vi "SP Get CH Controls.vi"(5 "S Parameter Test Parameters":T8={"Stimulus"={"Use Instrument Settings"=FALSE, "Blank Frequencies"=FALSE, "Sweep Type"=enum."Linear", "Sweep"={"Fstart"=500.0, "Fstop"=1500.0, "Units"=enum."MHz", "Points"=2}, "Power (dBm)"=999.0, "IFBW (Hz)"=-1.0, "Sweep Time (s)"=-1.0, "Calibration"={"State"=FALSE, "String"=""}}, "Measurement"={"Auto Select"=TRUE, "Data Source"=enum."VNA", "Ports"=2, "Parameters"=[]}, "De-Embed"={"De-Embed"=FALSE, "Adapters"=[]}, "Display"={"Lock Control"=FALSE, "Retain Settings"=TRUE, "Formatted Data"=FALSE, "Plot Orientation"=enum."Single", "Plot Controls"=[{"Trace Orientation"=enum."Overlay", "Frequency"={"Change Frequency"=FALSE, "Start"=500.0, "Stop"=1500.0, "Units"=enum."MHz"}, "Markers"=[], "Traces"=[]}, {"Trace Orientation"=enum."Overlay", "Frequency"={"Change Frequency"=FALSE, "Start"=500.0, "Stop"=1500.0, "Units"=enum."MHz"}, "Markers"=[], "Traces"=[]}, {"Trace Orientation"=enum."Overlay", "Frequency"={"Change Frequency"=FALSE, "Start"=500.0, "Stop"=1500.0, "Units"=enum."MHz"}, "Markers"=[], "Traces"=[]}, {"Trace Orientation"=enum."Overlay", "Frequency"={"Change Frequency"=FALSE, "Start"=500.0, "Stop"=1500.0, "Units"=enum."MHz"}, "Markers"=[], "Traces"=[]}]}, "Limits"=[], "Filter Limits"=[]} {"Filter Limits"."Parameter"."Stimulus Port" min=1 step=1; "Filter Limits"."Parameter"."Response Port" min=1 step=1; "Filter Limits"."Passband"."Bandwidth Attn" format="%.3g"; "Filter Limits"."Passband"."Stop/Span" format="%.3g"; "Filter Limits"."Passband"."Start/Center" format="%.3g"; "Measurement"."Parameters"."Channel" min=0 max=32 step=1; "Measurement"."Parameters"."Parameter"."Stimulus Port" min=1 step=1; "Measurement"."Parameters"."Parameter"."Response Port" min=1 step=1; "Limits"."Parameter"."Stimulus Port" min=1 step=1; "Limits"."Parameter"."Response Port" min=1 step=1; "Stimulus"."Sweep Time (s)" format="%.3g"; "Display"."Plot Controls"."Traces"."Reference" format="%#.2g"; "Display"."Plot Controls"."Traces"."Display Data" items=["Data", "Memory", "Data/Memory"]; "Display"."Plot Controls"."Traces"."Format" items=["Log Mag", "Phase", "Expanded Phase", "Delay", "Smith", "Polar", "Lin Mag", "SWR", "Loss", "Real", "Imaginary"]; "Display"."Plot Controls"."Traces"."Scale" min=0.001 step=1.0 format="%#.2g"; "Display"."Plot Controls"."Traces"."Position" min=0.0 max=10.0; "Display"."Plot Controls"."Frequency"."Stop" format="%.3g"; "Display"."Plot Controls"."Frequency"."Start" format="%.3g"}, 6 "Channel":i8=1, 7 "Plot Reference":refnum<vi>) -> (0 "Channel Control":T5={"Trace On"=TRUE, "Measure"=0, "Format"=0, "Autoscale"=TRUE, "Reference"=0.0, "\nRefUnit"="dB/Div", "Position"=5.0, "Scale"=10.0, "ScaleUnit"="dB/Div", "LimitOn"=TRUE, "LimitFill"=FALSE, "Display Data"=0, "Show Markers"=TRUE, "SXX"=""} {"Reference" format="%#.2g"; "Display Data" items=["Data", "Memory", "Data/Memory"]; "Format" items=["Log Mag", "Phase", "Expanded Phase", "Delay", "Smith", "Polar", "Lin Mag", "SWR", "Loss", "Real", "Imaginary"]; "Scale" min=0.001 step=1.0 format="%#.2g"; "Position" min=0.0 max=10.0}, 1 "CH Controls":T1={"Trace Orientation"=enum."Overlay", "Frequency"={"Change Frequency"=FALSE, "Start"=500.0, "Stop"=1500.0, "Units"=enum."MHz"}, "Markers"=[], "Traces"=[]} {"Traces"."Reference" format="%#.2g"; "Traces"."Display Data" items=["Data", "Memory", "Data/Memory"]; "Traces"."Format" items=["Log Mag", "Phase", "Expanded Phase", "Delay", "Smith", "Polar", "Lin Mag", "SWR", "Loss", "Real", "Imaginary"]; "Traces"."Scale" min=0.001 step=1.0 format="%#.2g"; "Traces"."Position" min=0.0 max=10.0; "Frequency"."Stop" format="%.3g"; "Frequency"."Start" format="%.3g"}, 4 "CH Controls Index":i8)   [LabVIEW 2011]
uses:
  TypeDefs/SP Display Trace Controls.ctl
  TypeDefs/SP Display Format.ctl
  TypeDefs/SP Display Data.ctl
  TypeDefs/SP Test Parameters.ctl
  TypeDefs/SP Stimulus Parameters.ctl
  TypeDefs/SP Frequency Units.ctl
  TypeDefs/SP Calibration State.ctl
  TypeDefs/SP Measurement.ctl
  TypeDefs/SP Parameters.ctl
  TypeDefs/SP Parameter.ctl
  TypeDefs/SP De-Embed.ctl
  TypeDefs/SP Adapter.ctl
  TypeDefs/SP Data.ctl
  TypeDefs/SP Display Parameters.ctl
  TypeDefs/SP Display Plot Controls Cluster.ctl
  TypeDefs/SP Marker Cluster.ctl
  TypeDefs/SP Marker Type.ctl
  TypeDefs/SP Limit.ctl
  TypeDefs/SP Format.ctl
  TypeDefs/SP Limit Type.ctl
  TypeDefs/SP Limit Point.ctl
  Test Referential Limit.ctl
  TypeDefs/SP Filter.ctl
  TypeDefs/SP Filter Type.ctl
  TypeDefs/SP Filter Passband.ctl
  TypeDefs/SP Frequency Format.ctl
  TypeDefs/SP Filter Ripple.ctl
  TypeDefs/SP Attenuation Point.ctl
  TypeDefs/SP Attenuation Type.ctl
  TypeDefs/SP Skirt Rejection Point.ctl
  TypeDefs/SP Relative Loss.ctl
panel:
  # "Div"
  # "Div"
  # "Div"
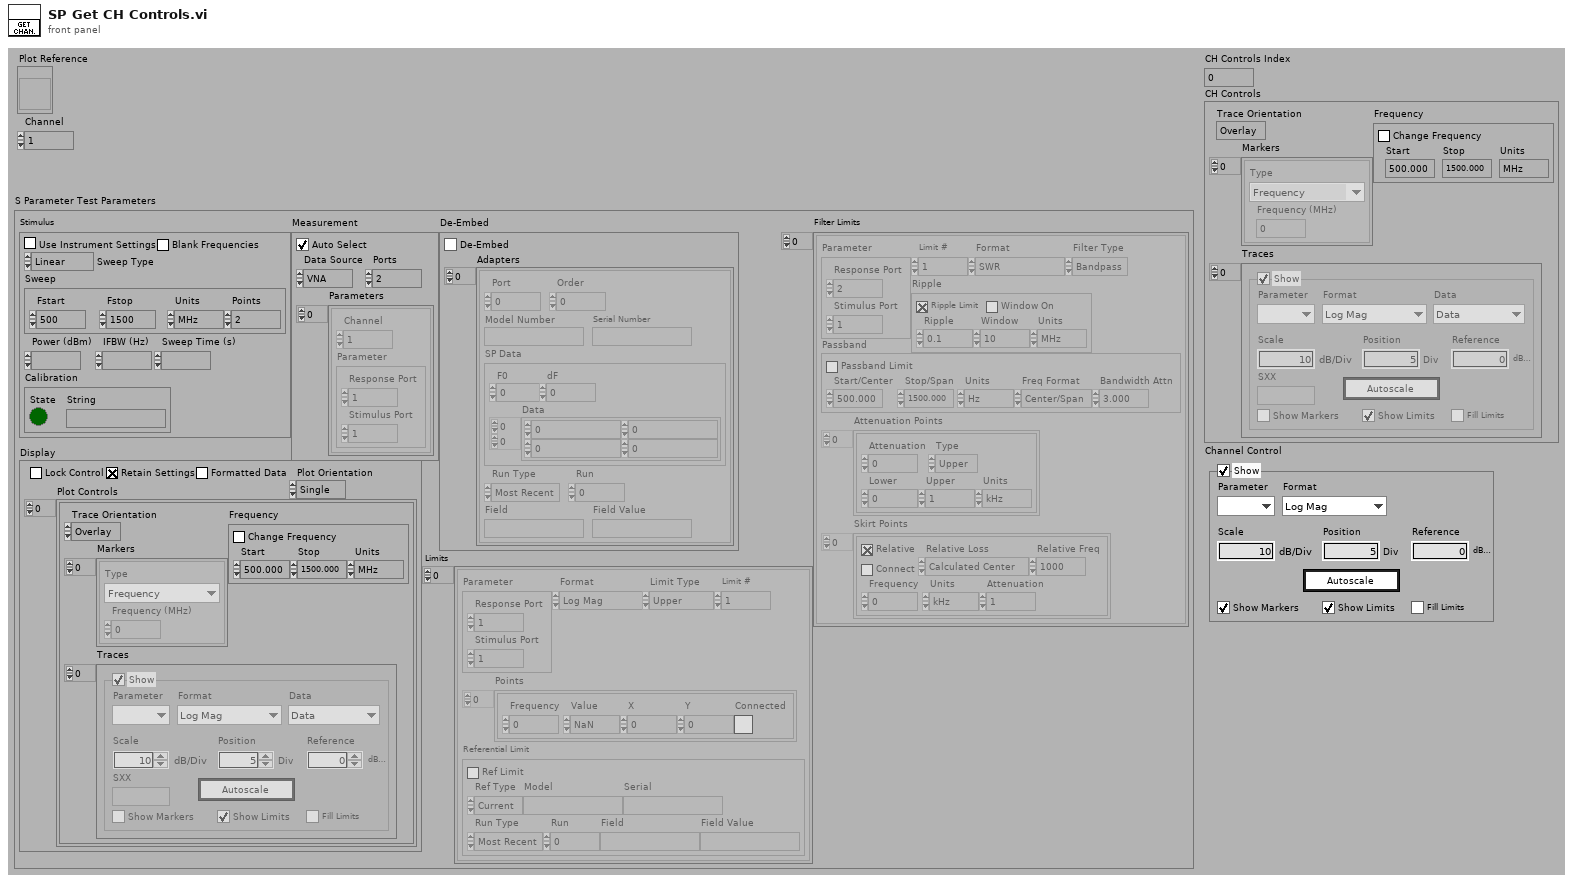
[diagram p1: front panel]
types:
  T1 = typedef "SP Display Plot Controls Cluster.ctl" = cluster{"Trace Orientation":enum32{"Overlay", "Split"}, "Frequency":cluster{"Change Frequency":bool, "Start":dbl, "Stop":dbl, "Units":T2}, "Markers":T3[], "Traces":T5[]}
  T2 = typedef "SP Frequency Units.ctl" = enum16{"Hz", "kHz", "MHz", "GHz", "Points"}
  T3 = typedef "SP Marker Cluster.ctl" = cluster{"Type":T4, "Frequency (MHz)":dbl}
  T4 = typedef "SP Marker Type.ctl" = enum16{"Frequency", "Trace Maximum", "Trace Minimum", "Limit Maximum", "Limit Minimum"}
  T5 = typedef "SP Display Trace Controls.ctl" = cluster{"Trace On":bool, "Measure":i32, "Format":T6, "Autoscale":bool, "Reference":dbl, "\nRefUnit":string, "Position":dbl, "Scale":dbl, "ScaleUnit":string, "LimitOn":bool, "LimitFill":bool, "Display Data":T7, "Show Markers":bool, "SXX":string}
  T6 = typedef "SP Display Format.ctl" = i32
  T7 = typedef "SP Display Data.ctl" = u16
  T8 = typedef "SP Test Parameters.ctl" = cluster{"Stimulus":T9, "Measurement":T11, "De-Embed":T14, "Display":T17, "Limits":T18[], "Filter Limits":T23[]}
  T9 = typedef "SP Stimulus Parameters.ctl" = cluster{"Use Instrument Settings":bool, "Blank Frequencies":bool, "Sweep Type":enum32{"Linear", "Logarithmic", "List", "Power", "CW"}, "Sweep":cluster{"Fstart":dbl, "Fstop":dbl, "Units":T2, "Points":i32}, "Power (dBm)":dbl, "IFBW (Hz)":dbl, "Sweep Time (s)":dbl, "Calibration":T10}
  T10 = typedef "SP Calibration State.ctl" = cluster{"State":bool, "String":string}
  T11 = typedef "SP Measurement.ctl" = cluster{"Auto Select":bool, "Data Source":enum16{"VNA", "Data File"}, "Ports":i8, "Parameters":T12[]}
  T12 = typedef "SP Parameters.ctl" = cluster{"Channel":i8, "Parameter":T13}
  T13 = typedef "SP Parameter.ctl" = cluster{"Stimulus Port":i8, "Response Port":i8}
  T14 = typedef "SP De-Embed.ctl" = cluster{"De-Embed":bool, "Adapters":T15[]}
  T15 = typedef "SP Adapter.ctl" = cluster{"Port":i8, "Order":i8, "Model Number":string, "Serial Number":string, "SP Data":T16, "Run Type":enum16{"Most Recent", "Run #", "Match Field"}, "Run":i32, "Field":string, "Field Value":string}
  T16 = typedef "SP Data.ctl" = cluster{"F0":dbl, "dF":dbl, "Data":cdb[][]}
  T17 = typedef "SP Display Parameters.ctl" = cluster{"Lock Control":bool, "Retain Settings":bool, "Formatted Data":bool, "Plot Orientation":enum32{"Single", "Dual", "Quad"}, "Plot Controls":T1[]}
  T18 = typedef "SP Limit.ctl" = cluster{"Parameter":T13, "Format":T19, "Limit Type":T20, "Points":T21[], "Referential Limit":T22, "Limit #":i8}
  T19 = typedef "SP Format.ctl" = enum16{"Log Mag", "Lin Mag", "SWR", "Phase", "Expanded Phase", "Delay", "Insertion Loss", "Isolation", "Return Loss"}
  T20 = typedef "SP Limit Type.ctl" = enum16{"Upper", "Lower", "Delta", "Filter", "Referential"}
  T21 = typedef "SP Limit Point.ctl" = cluster{"Frequency":dbl, "Value":dbl, "X":dbl, "Y":dbl, "Connected":bool}
  T22 = typedef "Test Referential Limit.ctl" = cluster{"Ref Limit":bool, "Ref Type":enum16{"Current", "Specify"}, "Model":string, "Serial":string, "Run Type":enum16{"Most Recent", "Run #", "Match Field"}, "Run":i32, "Field":string, "Field Value":string}
  T23 = typedef "SP Filter.ctl" = cluster{"Limit #":i8, "Parameter":T13, "Format":T19, "Filter Type":T24, "Passband":T25, "Ripple":T27, "Attenuation Points":T28[], "Skirt Points":T30[]}
  T24 = typedef "SP Filter Type.ctl" = enum16{"Lowpass", "Highpass", "Bandpass", "Bandstop"}
  T25 = typedef "SP Filter Passband.ctl" = cluster{"Start/Center":dbl, "Stop/Span":dbl, "Units":T2, "Freq Format":T26, "Bandwidth Attn":dbl, "Passband Limit":bool}
  T26 = typedef "SP Frequency Format.ctl" = enum16{"Start/Stop", "Center/Span"}
  T27 = typedef "SP Filter Ripple.ctl" = cluster{"Ripple Limit":bool, "Window On":bool, "Ripple":dbl, "Window":dbl, "Units":T2}
  T28 = typedef "SP Attenuation Point.ctl" = cluster{"Attenuation":dbl, "Type":T29, "Lower":dbl, "Upper":dbl, "Units":T2}
  T29 = typedef "SP Attenuation Type.ctl" = enum16{"Center", "Lower", "Upper"}
  T30 = typedef "SP Skirt Rejection Point.ctl" = cluster{"Relative":bool, "Connect":bool, "Frequency":dbl, "Units":T2, "Attenuation":dbl, "Relative Loss":T31, "Relative Freq":dbl}
  T31 = typedef "SP Relative Loss.ctl" = enum16{"Calculated Center", "Passband Minimum", "Passband Maximum", "Passband Average", "Frequency"}
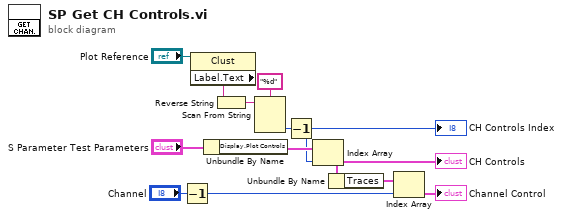
[diagram p0: block diagram]
diagram:
  n1 = Decrement(x="Channel") -> (x-1=w2:i8)
  n2 = property class="Clust"(reference="Plot Reference") -> ("Label.Text"=w12:string)  [unwired: 1 in, 2 out]
  n3 = Unbundle By Name("S Parameter Test Parameters") -> ("Display.Plot Controls"=w8:T1[])
  n4 = Reverse String(1:w12) -> (0:w11:string)
  n5 = Scan From String(format string="%d", input string=w11) -> (output 1=w7:i32)  [unwired: 2 in, 4 out]
  n6 = Decrement(x=w7) -> (x-1=w6:i32)
  "CH Controls Index" <- w6
  n7 = Index Array(array=w8, index=w6) -> (element=w5:T1)
  "CH Controls" <- w5
  n8 = Unbundle By Name(w5) -> ("Traces"=w4:T5[])
  n9 = Index Array(array=w4, index=w2) -> (element=→"Channel Control":T5)
